vi "InitDGSystem and HW.vi"(6 "InitHW(false)":bool, 7 "System":T1, 8 "error in":errorcluster, 9 "Chnls":T9[](array[typedef]) {"ChnParameter"."Delay (µs)" min=0.0 max=100000000.0 format="%.4f"; "G08_Chnl_Settings"."Pulse Width (µs)" min=0.0 max=8947840.0 format="%#.6f"; "Go and Done Signal"."Done Signal" format="%04x" items=["Local Primary"=1, "Local Secondary"=2, "Local Force"=4, "Master Primary"=16]; "Go and Done Signal"."Go Signal" format="%04x" items=["Local Primary0x1"=1, "Local Secondary0x2"=2, "Local Force 0x4"=4, "Resynchronize 0x8"=8, "Master Prim. 0x10"=16, "Master Sec. 0x20"=32, "Master Force  0x40"=64, "System Clock 0x80"=128, "Delay Clock 0x100"=256, "Inhibit Local 0x200"=512, "Start Local 0x400"=1024, "Start Bus 0x800"=2048, "Step Back Local 0x1000"=4096, "Step Back Bus 0x2000"=8192, "RunCircle 0x4000"=16384, "SyncReload 0x8000"=32768, "From E 0x10000"=65536, "From F 0x20000"=131072, "From Bus 0x40000"=262144]}, 10 "Cards":T3[](array[typedef]) {"Advanced Settings"."Trigger on MS Bus" format="%04x" items=["Local Primary0x1"=1, "Local Secondary0x2"=2, "Local Force 0x4"=4, "Resynchronize 0x8"=8, "StepBackOnBus 0x10"=16, "StartOnBus 0x20"=32, "InhibitOnBus 0x40"=64, "LoadDataOnBus 0x80"=128]; "Advanced Settings"."Force Trigger (µs)" min=0.0 format="%.6f"; "SG08_Settings"."StepBackTime (µs)" min=0.0 format="%.6f"; "SG08_Settings"."Gate Delay (µs)" format="%.3f"; "SG08_Settings"."Gate Level" min=-2.5 max=2.5 format="%.3g"; "Base Settings"."Gate Divider" min=1 max=1000000; "Base Settings"."Clock Source" items=["Internal Oscillator"=1, "External Trigger"=2, "Trigger-> Oscillator"=3, "MasterSlave Bus"=4]; "Base Settings"."Inhibit(µs)" format="%#_11g"}, 11 "BME_DG_System in":refnum<class "BME_DG_System.lvclass">) -> (0 "error out":errorcluster, 2 "Problem Chnls out":string[](array[string]), 3 "BME_DG_System in":refnum<class "BME_DG_System.lvclass">)   [LabVIEW 2009, in "POLARIS BME DG.lvlib" / "BME_DG_System.lvclass"]
uses:
  BME_DG_System.lvclass
  Chnl Settings Complete.ctl
  LV-BME Interface/ChnlSettings.ctl
  Go_Done_Chnl_Settings.ctl
  GoSignalBits.ctl
  SG08_Chnl_Settings.ctl
  Card Config.ctl
  LV-BME Interface/BME_DG_TriggerSettings.ctl
  LV-BME Interface/ClockSource.ctl
  SG08_Settings.ctl
  LV-BME Interface/BME_DG_V2TriggerSettings.ctl
  MSBusSignals.ctl
  System DG Selection.ctl
  DetectDG.ctl
  BME_DG_System.lvclass/BME_DG_System.ctl
  BME_DG_Base/BME_DG_Base.lvclass
  BME_DG_Chnl/BME_DG_Chnl.lvclass
  POLARIS BME DG.lvlib
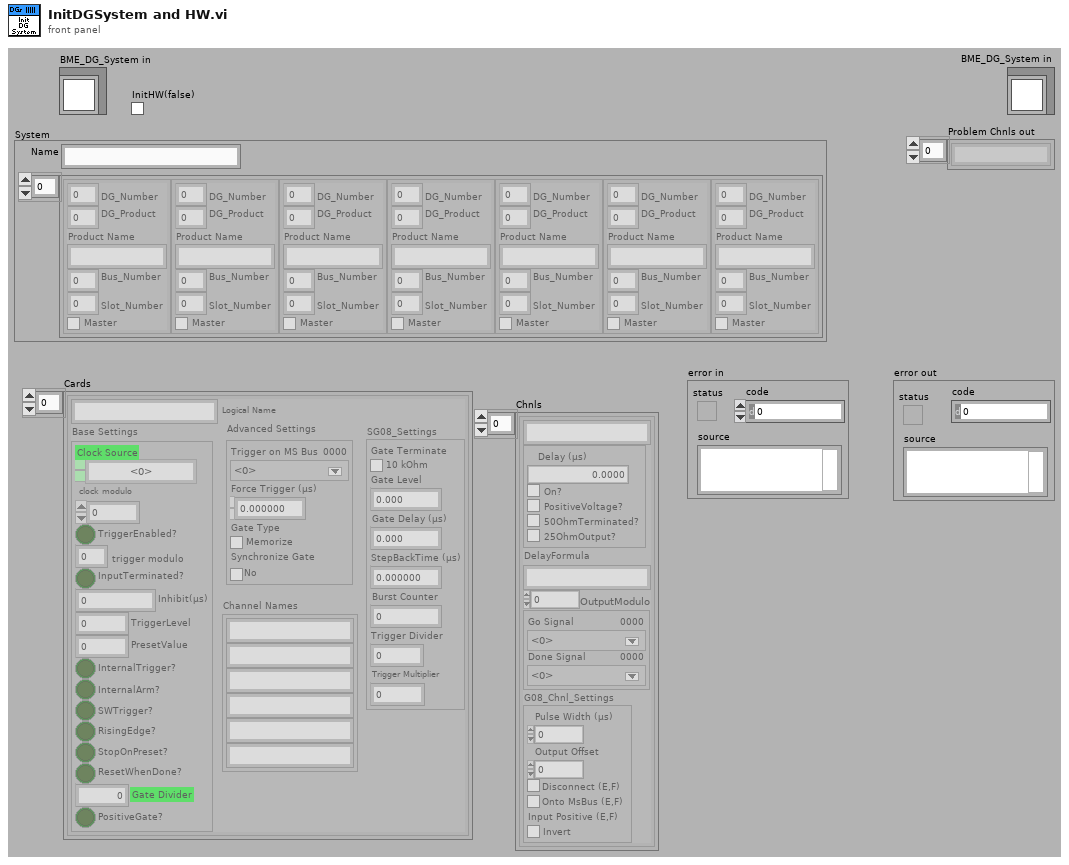
[diagram p1: front panel]
types:
  T1 = typedef "POLARIS BME DG.lvlib/System DG Selection.ctl" = cluster{"Selected System DGs":T2[], "Name":string}
  T2 = typedef "POLARIS BME DG.lvlib/DetectDG.ctl" = cluster{"DG_Number":i32, "DG_Product":i32, "Product Name":string, "Bus_Number":i32, "Slot_Number":i32, "Master":bool}
  T3 = typedef "POLARIS BME DG.lvlib/Card Config.ctl" = cluster{"Logical Name":string, "Base Settings":T4, "SG08_Settings":T6, "Channel Names":string[], "Advanced Settings":T7}
  T4 = typedef "POLARIS BME DG.lvlib/BME_DG_TriggerSettings.ctl" = cluster{"Clock Source":T5, " clock modulo":u32, "TriggerEnabled?":bool, "trigger modulo ":i32, "InputTerminated?":bool, "Inhibit(µs)":dbl, "TriggerLevel":dbl, "PresetValue":i32, "InternalTrigger?":bool, "InternalArm?":bool, "SWTrigger?":bool, "RisingEdge?":bool, "StopOnPreset?":bool, "ResetWhenDone?":bool, "Gate Divider":i32, "PositiveGate?":bool}
  T5 = typedef "POLARIS BME DG.lvlib/ClockSource.ctl" = i32
  T6 = typedef "POLARIS BME DG.lvlib/SG08_Settings.ctl" = cluster{"Gate Terminate":bool, "Gate Level":dbl, "Gate Delay (µs)":dbl, "StepBackTime (µs)":dbl, "Burst Counter":u32, "Trigger Divider":u32, "Trigger Multiplier":u32}
  T7 = typedef "POLARIS BME DG.lvlib/BME_DG_V2TriggerSettings.ctl" = cluster{"Trigger on MS Bus":T8, "Force Trigger (µs)":dbl, "Gate Type":bool, "Synchronize Gate":bool}
  T8 = typedef "POLARIS BME DG.lvlib/MSBusSignals.ctl" = u32
  T9 = typedef "POLARIS BME DG.lvlib/Chnl Settings Complete.ctl" = cluster{"Channel Name":string, "ChnParameter":T10, "DelayFormula":string, "OutputModulo":i32, "Go and Done Signal":T11, "G08_Chnl_Settings":T13}
  T10 = typedef "POLARIS BME DG.lvlib/ChnlSettings.ctl" = cluster{" Delay (µs)":dbl, "On?":bool, "PositiveVoltage?":bool, "50OhmTerminated? ":bool, "25OhmOutput?":bool}
  T11 = typedef "POLARIS BME DG.lvlib/Go_Done_Chnl_Settings.ctl" = cluster{"Go Signal":T12, "Done Signal":u32}
  T12 = typedef "POLARIS BME DG.lvlib/GoSignalBits.ctl" = u32
  T13 = typedef "POLARIS BME DG.lvlib/SG08_Chnl_Settings.ctl" = cluster{"Pulse Width (µs)":dbl, "Output Offset":u32, "Disconnect (E,F)":bool, "Onto MsBus (E,F)":bool, "Input Positive (E,F)":bool}
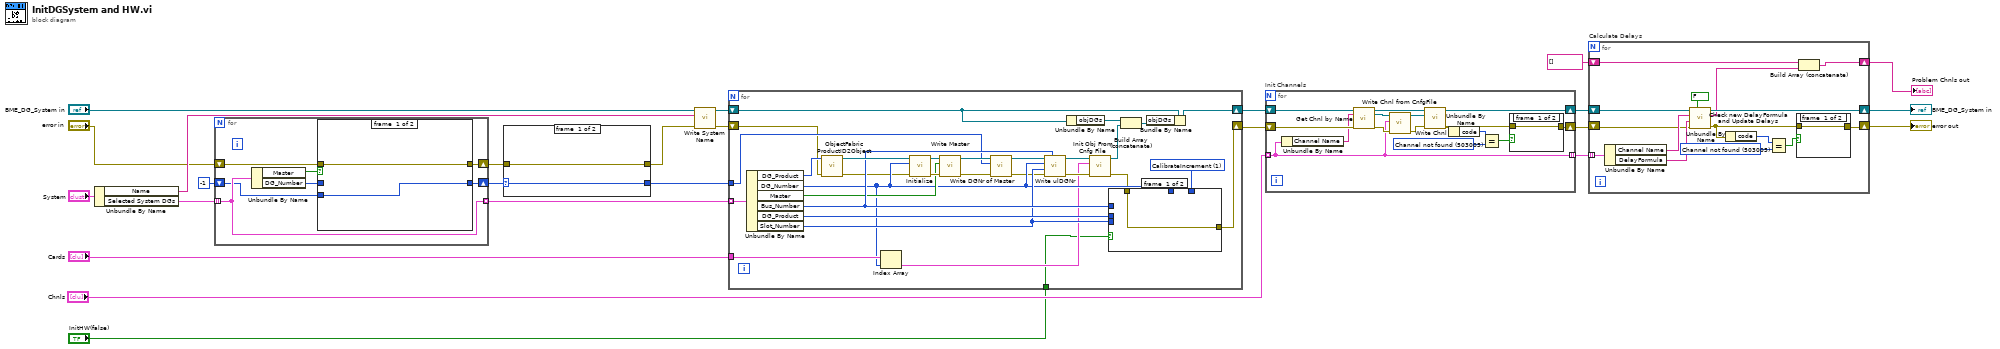
[diagram p0: block diagram]
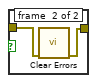
[diagram p2: hidden frame]
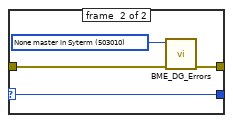
[diagram p3: hidden frame]
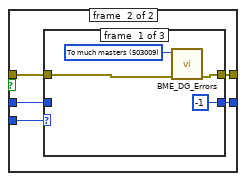
[diagram p4: hidden frame]
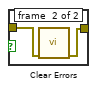
[diagram p7: hidden frame]
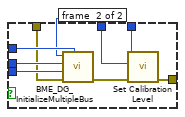
[diagram p8: hidden frame]
diagram:
  n1 = Unbundle By Name("System") -> ("Name"=w14:string, "Selected System DGs"=w11:T2[])
  n2 = for {
    tunnel: w11 -> [w32] mode=indexing
    tunnel: [w32] -> w10 mode=indexing
    shift-right: [w29] -> w5
    shift-left: -1 ("DG_Number") -> [w30]
    shift-right: [w26] -> w7
    shift-left: "error in" -> [w27]
    n3 = Unbundle By Name(w32) -> ("Master"=w31:bool, "DG_Number"=w28:i32)
    n4 = case shown="True" w31 {
      tunnel: w30 -> [w34 w39]
      tunnel: [w34 w38] -> w29
      tunnel: w28 -> [_ w37]
      tunnel: w27 -> [w33 w36]
      tunnel: [w33 w35] -> w26
      frame #0 {
      }
      frame #1 {
        n5 = case shown="0, Default" w39 {
          selector: w39 -> [_ w45 _]
          tunnel: [-1 ("DG_Number") w45 w47] -> w38
          tunnel: w37 -> [_ _ w47]
          tunnel: w36 -> [w42 w44 w46]
          tunnel: [w41 w44 w46] -> w35
          frame #0 {
            w40 = 503009 items=["Channel refers itself"=503001, "Deadloop"=503002, "Negative Delay"=503003, "Delay Card not found"=503004, "Channel not found"=503005, "Parse Error"=503006, "Not Supported"=503007, "Systen not found"=503008, "To much masters"=503009, "None master in Syterm"=503010] ("error")
            n6 = call "BME_DG_Errors.vi"("error in (no error)"=w42, "error"=w40) -> ("error out"=w41:errorcluster)  [unwired: 9 in]
          }
          frame #1 {
          }
          frame #2 {
          }
        }
      }
    }
  }
  n7 = case shown="-1" w5 {
    selector: w5 -> [w48 w50]
    tunnel: w7 -> [w49 w53]
    tunnel: [w49 w52] -> w6
    tunnel: [w48 w50] -> w4
    frame #0 {
    }
    frame #1 {
      w51 = 503010 items=["Channel refers itself"=503001, "Deadloop"=503002, "Negative Delay"=503003, "Delay Card not found"=503004, "Channel not found"=503005, "Parse Error"=503006, "Not Supported"=503007, "Systen not found"=503008, "To much masters"=503009, "None master in Syterm"=503010] ("error")
      n8 = call "BME_DG_Errors.vi"("error in (no error)"=w53, "error"=w51) -> ("error out"=w52:errorcluster)  [unwired: 9 in]
    }
  }
  n9 = call "Write System Name.vi"("error in (no error)"=w6, "log Name"=w14, "BME_DG_System in"="BME_DG_System in") -> ("error out"=w13:errorcluster, "BME_DG_System out"=w15:refnum<class "BME_DG_System.lvclass">)  [unwired: 7 in]
  n10 = for {
    tunnel: w10 -> [w76] mode=indexing
    shift-right: [w83] -> w19
    shift-left: w15 -> [w82]
    tunnel: "Cards" -> [w68]
    shift-right: [w70] -> w20
    shift-left: w13 -> [w55]
    tunnel: w4 -> [w59]
    tunnel: "InitHW(false)" -> [w56]
    w69 = u32 1 items=["None", "CalibrateIncrement", "CalibrateOffset"] ("CalibrationLevel")
    n11 = Unbundle By Name(w76) -> ("DG_Product"=w73:i32, "DG_Number"=w67:i32, "Master"=w74:bool, "Bus_Number"=w75:i32, "DG_Product"=w72:i32, "Slot_Number"=w71:i32)
    n12 = call "ObjectFabric ProductID2Object.vi"("error in (no error)"=w55, "DG_Product"=w73) -> ("error out"=w54:errorcluster, "BME_DG_Base"=w79:refnum<class "BME_DG_Base.lvclass">)  [unwired: 7 in, 1 out]
    n13 = Index Array(array=w68, index=w67) -> (element=w64:T3)
    n14 = call-dynamic "Initialize.vi"("error in (no error)"=w54, "DG Nr"=w67, "BME_DG_Base in"=w79) -> ("error out"=w78:errorcluster, "BME_DG_Base out"=w77:refnum<class "BME_DG_Base.lvclass">)  [unwired: 7 in]
    n15 = call-dynamic "Write Master.vi"("error in (no error)"=w78, "Master?"=w74, "BME_DG_Base in"=w77) -> ("error out"=w58:errorcluster, "BME_DG_Base out"=w61:refnum<class "BME_DG_Base.lvclass">)  [unwired: 7 in]
    n16 = call-dynamic "Write DGNr of Master.vi"("error in (no error)"=w58, "DGNr of Master"=w59, "BME_DG_Base in"=w61) -> ("error out"=w57:errorcluster, "BME_DG_Base out"=w60:refnum<class "BME_DG_Base.lvclass">)  [unwired: 7 in]
    n17 = call-dynamic "Write ulDGNr.vi"("PCI BusNr"=w75, "error in (no error)"=w57, "ulSlotNr"=w71, "ulDGNr"=w67, "BME_DG_Base in"=w60) -> ("error out"=w65:errorcluster, "BME_DG_Base out"=w66:refnum<class "BME_DG_Base.lvclass">)  [unwired: 5 in]
    n18 = Unbundle By Name(w82) -> ("objDGs"=w80:refnum<class "BME_DG_Base.lvclass">[])
    n19 = call-dynamic "Init Obj From Cnfg File.vi"("error in (no error)"=w65, "Card Config"=w64, "BME_DG_Base in"=w66) -> ("error out"=w62:errorcluster, "BME_DG_Base out"=w63:refnum<class "BME_DG_Base.lvclass">)  [unwired: 7 in]
    n20 = case shown="True" w56 {
      tunnel: w75 -> [_ w92]
      tunnel: w72 -> [_ w91]
      tunnel: w71 -> [_ w90]
      tunnel: [w84 w89] -> w70
      tunnel: w69 -> [_ w88]
      tunnel: w67 -> [_ w87]
      tunnel: w62 -> [w84 w86]
      frame #0 {
      }
      frame #1 {
        n21 = call "BME_DG_InitializeMultipleBus.vi"("BusNr"=w92, "error in (no error)"=w86, "Slot Number"=w90, "DG_Product"=w91, "DG_Number"=w87) -> ("error out"=w85:errorcluster)  [unwired: 5 in]
        n22 = call "Set Calibration Level.vi"("error in (no error)"=w85, "DG Number"=w87, "CalibrationLevel"=w88) -> ("error out"=w89:errorcluster)  [unwired: 8 in]
      }
    }
    n23 = Build Array (concatenate)(w80, w63) -> (w81:refnum<class "BME_DG_Base.lvclass">[])
    n24 = Bundle By Name(cluster=w82, "objDGs"=w81) -> (w83:refnum<class "BME_DG_System.lvclass">)
  }
  n25 = for "Init Channels" {
    tunnel: "Chnls" -> [w99] mode=indexing
    shift-right: [w105] -> w24
    shift-left: w19 -> [w107]
    shift-right: [w95] -> w25
    shift-left: w20 -> [w106]
    tunnel: [w99] -> w23 mode=indexing
    w98 = 503005 items=["Channel refers itself"=503001, "Deadloop"=503002, "Negative Delay"=503003, "Delay Card not found"=503004, "Channel not found"=503005, "Parse Error"=503006, "Not Supported"=503007, "Systen not found"=503008] ("error")
    n26 = Unbundle By Name(w99) -> ("Channel Name"=w93:string)
    n27 = call "Get Chnl by Name.vi"("BME_DG_System in"=w107, "Chnl Name"=w93, "error in (no error)"=w106) -> ("BME_DG_System out"=w104:refnum<class "BME_DG_System.lvclass">, "BME_DG_Chnl"=w103:refnum<class "BME_DG_Chnl.lvclass">, "error out"=w101:errorcluster)  [unwired: 7 in, 3 out]
    n28 = call-dynamic "Write Chnl from CnfgFile.vi"("error in (no error)"=w101, "ChnlSettings"=w99, "BME_DG_Chnl in"=w103) -> ("error out"=w100:errorcluster, "BME_DG_Chnl out"=w102:refnum<class "BME_DG_Chnl.lvclass">)  [unwired: 7 in]
    n29 = call "Write Chnl.vi"("error in (no error)"=w100, "BME_DG_Chnl.lvclass"=w102, "BME_DG_System in"=w104) -> ("error out"=w96:errorcluster, "BME_DG_System out"=w105:refnum<class "BME_DG_System.lvclass">)  [unwired: 7 in]
    n30 = Unbundle By Name(w96) -> ("code"=w97:i32)
    n31 = Equal?(x=w97, y=w98) -> (x = y?=w94:bool)
    n32 = case shown="True" w94 {
      tunnel: w96 -> [w108 w110]
      tunnel: [w108 w109] -> w95
      frame #0 {
      }
      frame #1 {
        n33 = call <vilib>:"Clear Errors.vi"("error in (no error)"=w110) -> ("error out"=w109:errorcluster)  [unwired: 6 in]
      }
    }
  }
  n34 = for "Calculate Delays" {
    shift-right: [w123] -> w21
    shift-left: w24 -> [w125]
    shift-right: [w116] -> w22
    shift-left: w25 -> [w114]
    tunnel: w23 -> [w122] mode=indexing
    shift-right: [w112] -> w3
    shift-left: string[] [] ("Problem Chnls out") -> [w111]
    w117 = 503005 items=["Channel refers itself"=503001, "Deadloop"=503002, "Negative Delay"=503003, "Delay Card not found"=503004, "Channel not found"=503005, "Parse Error"=503006, "Not Supported"=503007, "Systen not found"=503008] ("error")
    n35 = Unbundle By Name(w122) -> ("Channel Name"=w121:string, "DelayFormula"=w120:string)
    n36 = call "Check new DelayFormula and Update Delays.vi"("Update HW"=FALSE, "error in (no error)"=w114, "Delay Formula"=w120, "ChnlName"=w121, "BME_DG_System in"=w125) -> ("error out"=w115:errorcluster, "Problem Chnls out"=w113:string[], "BME_DG_System out"=w123:refnum<class "BME_DG_System.lvclass">)  [unwired: 3 in, 1 out]
    n37 = Unbundle By Name(w115) -> ("code"=w118:i32)
    n38 = Equal?(x=w118, y=w117) -> (x = y?=w119:bool)
    n39 = case shown="True" w119 {
      tunnel: w115 -> [w126 w128]
      tunnel: [w126 w127] -> w116
      frame #0 {
      }
      frame #1 {
        n40 = call <vilib>:"Clear Errors.vi"("error in (no error)"=w128) -> ("error out"=w127:errorcluster)  [unwired: 6 in]
      }
    }
    n41 = Build Array (concatenate)(w111, w113) -> (w112:string[])
  }
  "error out" <- w22
  "BME_DG_System in" <- w21
  "Problem Chnls out" <- w3
